vi "接收消息解析.vi"(11 "上位机消息":string) -> (0 "状态":i32, 1 "角度":dbl, 2 "Y":i32, 3 "X":i32)   [LabVIEW 2016]
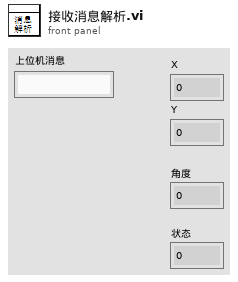
[diagram p1: front panel]
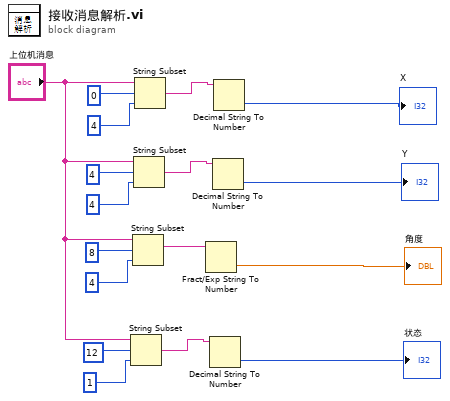
[diagram p0: block diagram]
diagram:
  n1 = String Subset(string="上位机消息", offset (0)=12, length (rest)=1) -> (substring=w7:string)
  n2 = String Subset(string="上位机消息", offset (0)=8, length (rest)=4) -> (substring=w4:string)
  n3 = String Subset(string="上位机消息", offset (0)=4, length (rest)=4) -> (substring=w14:string)
  n4 = String Subset(string="上位机消息", offset (0)=0, length (rest)=4) -> (substring=w15:string)
  n5 = Fract/Exp String To Number(string=w4) -> (number=→"角度":dbl)  [unwired: 3 in, 1 out]
  n6 = Decimal String To Number(string=w7) -> (number=→"状态":i32)  [unwired: 2 in, 1 out]
  n7 = Decimal String To Number(string=w14) -> (number=→"Y":i32)  [unwired: 2 in, 1 out]
  n8 = Decimal String To Number(string=w15) -> (number=→"X":i32)  [unwired: 2 in, 1 out]
